vi "Verify Analog Waveform in LV.vi"(4 "a1":string, 5 "a2":T1, 6 "Y":dbl[](array[numeric]), 7 "dt":dbl, 8 "t0":timestamp, 9 "waveform in":waveform(dbl)={"t0"=timestamp(0 s since 1904-01-01), "dt"=0.0, "Y"=[]}) -> (0 "a2 equal":bool, 1 "a1 equal":bool, 2 "Components equal":bool, 3 "waveform out":waveform(dbl))   [LabVIEW 2013]
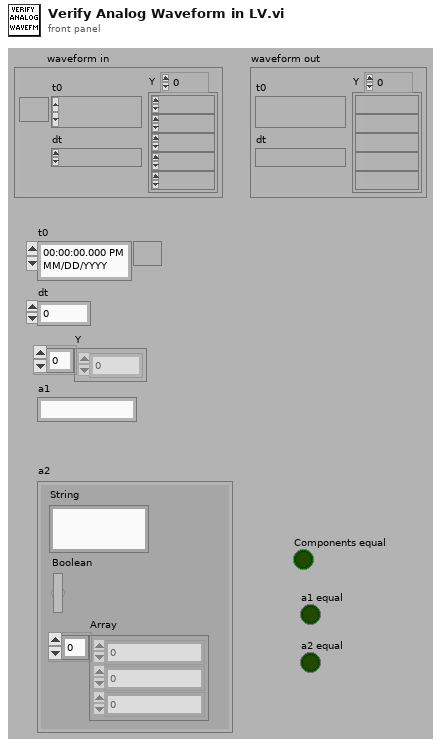
[diagram p1: front panel]
types:
  T1 = cluster{"String":string, "Boolean":bool, "Array":cxt[]}
  T2 = cluster{"String":bool, "Boolean":bool, "Array":bool[]}
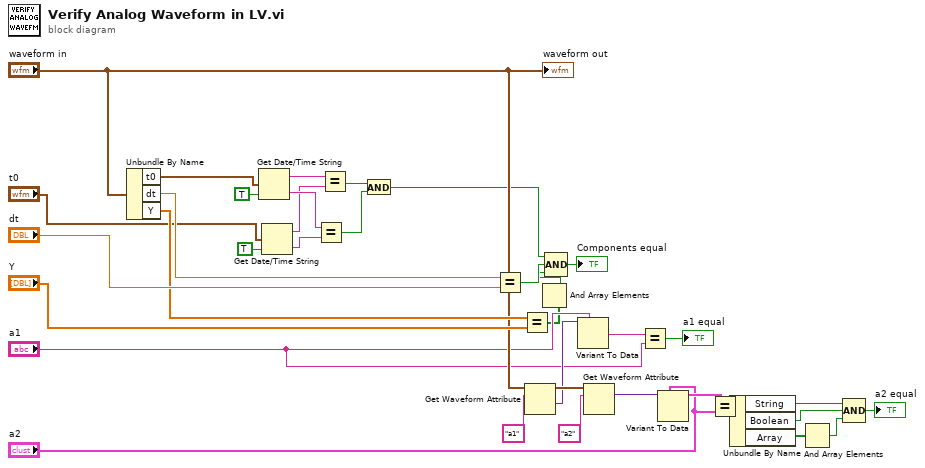
[diagram p0: block diagram]
diagram:
  n1 = Unbundle By Name("waveform in") -> ("t0"=w2:timestamp, "dt"=w36:dbl, "Y"=w34:dbl[])
  n2 = Get Date/Time String(seconds (now)=w2, want seconds? (F)=TRUE) -> (date string=w6:string, time string=w9:string)  [unwired: 1 in]
  n3 = Get Date/Time String(seconds (now)="t0", want seconds? (F)=TRUE) -> (date string=w7:string, time string=w8:string)  [unwired: 1 in]
  n4 = Equal?(x=w9, y=w8) -> (x = y?=w5:bool)
  n5 = Equal?(x=w6, y=w7) -> (x = y?=w4:bool)
  n6 = And(x=w4, y=w5) -> (x .and. y?=w3:bool)
  n7 = Equal?(x=w36, y="dt") -> (x = y?=w15:bool)
  n8 = Equal?(x=w34, y="Y") -> (x = y?=w14:bool[])
  n9 = Get Waveform Attribute(6:"a1" ("name"), 7:"waveform in") -> (1:w28:variant, 3:w30:waveform(dbl))  [unwired: 2 in, 2 out]
  n10 = And Array Elements(Boolean array=w14) -> (logical AND=w13:bool)
  n11 = Compound Arithmetic op=AND(w3, w15, w13) -> (→"Components equal":bool)
  n12 = Variant To Data(type="a1", Variant=w28) -> (data=w27:string)  [unwired: 1 in, 1 out]
  n13 = Get Waveform Attribute(6:"a2" ("name"), 7:w30) -> (1:w25:variant)  [unwired: 2 in, 3 out]
  n14 = Equal?(x=w27, y="a1") -> (x = y?=→"a1 equal":bool)
  n15 = Variant To Data(type="a2", Variant=w25) -> (data=w24:T1)  [unwired: 1 in, 1 out]
  n16 = Equal?(x=w24, y="a2") -> (x = y?=w21:T2)
  n17 = Unbundle By Name(w21) -> ("String"=w17:bool, "Boolean"=w18:bool, "Array"=w20:bool[])
  n18 = And Array Elements(Boolean array=w20) -> (logical AND=w19:bool)
  n19 = Compound Arithmetic op=AND(w17, w18, w19) -> (→"a2 equal":bool)
  "waveform out" <- "waveform in"
